vi "PH_Timing.get Timing Mode.vi"(0 "i ref in":refnum<vi>, 5 "error in":errorcluster) -> (14 "i ref out":refnum<vi>, 19 "error out":errorcluster)   [LabVIEW 2014, in "PH_Timing.lvlib"]
doc: "This VI calculates the information concerning the timing mode, writes them to own attributtes and publishes the information."
uses:
  PH_Timing.lvlib
  lib.lib/DimLVEvent/LVDimInterface/LVDimInterface.lvlib
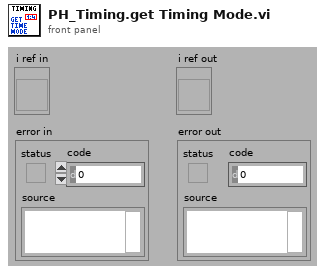
[diagram p1: front panel]
types:
  T1 = typedef "PH_Timing.lvlib/PH_Timing.i attribute.ctl" = cluster{"Sequencer":cluster{"linked?":bool, "Proc State":string, "Ref State":refnum<vi>}, "Gate Generator":cluster{"GD":cluster{"Device Status":T2, "linked?":bool}, "Settings":T3, "GUI Ref":refnum<vi>}, "Interlock Bypass":cluster{"Instancename":string, "Switch linked?":bool, "Device Status":T2, "Ref Status":refnum<vi>}, "Roughtuner":cluster{"Settings":T4, "GUI Ref":refnum<vi>, "GD":cluster{"Device Status":T2, "linked?":bool}}, "0,5Hz Gater":cluster{"Settings":T5, "GUI Ref":refnum<vi>, "GD":cluster{"Device Status":T2, "linked?":bool}}, "Slow Trigger":cluster{"Settings":T6, "GUI Ref":refnum<vi>, "Service ID Delay":i32, "Service ID Ext Trig":i32, "Wanted Settings":T6}, "Timing Mode":cluster{"Mode":T7, "GUI Ref":refnum<vi>, "Service ID T2":i32, "Service ID Mode":i32, "Wanted Mode":T7}, "ns Generator":cluster{"Settings":T8, "ns Generator Settings":refnum<vi>, "GD":cluster{"Device Status":T2, "linked?":bool}}, "Phase FEs":cluster{"Settings":T11, "GUI Ref":refnum<vi>, "Service ID Phase":i32, "Wanted Settings":T11}, "GD GUI Refs":refnum<vi>[], "Heads":T12[], "GUI Ref Delete":refnum<vi>}
  T2 = typedef "PH_StatusHandler.lvlib/PH_StatusHandler.Status.ctl" = i16
  T3 = typedef "PH_Timing.lvlib/PH_Timing.GateGen.ctl" = cluster{"Instance":string, "Channel Gate":i32, "Channel T2":i32, "Width Gate":dbl, "Width T2":dbl, "Delay Gate":dbl, "Delay T2":dbl, "Gate activ":bool, "T2 activ":bool, "System Mode":enum16{"Normal", "Single", "Burst", "Duty Cycle"}}
  T4 = typedef "PH_Timing.lvlib/PH_Timing.Roughtuner.ctl" = cluster{"Instance":string, "Phase PHELIX / UNILAC":cluster{"Channel":u16, "relative to":u16, "Delay [ms]":dbl}, "Pulse Length":cluster{"Channel":u16, "relative to":u16, "Delay [ms]":dbl}, "Trigger":cluster{"externally?":bool, "Rate [Hz]":dbl}}
  T5 = typedef "PH_Timing.lvlib/PH_Timing.0.5HzGater.ctl" = cluster{"Instance":string, "Channel ns FE Delay":i32, "Channel 0.5Hz":i32, "Width ns FE Delay":dbl, "Width 0.5Hz":dbl, "Delay ns FE Delay":dbl, "Delay 0.5Hz":dbl, "ns FE Delay active":bool, "0.5Hz activ":bool, "ns FE Delay inverted":bool, "0.5Hz inverted":bool}
  T6 = typedef "PH_Timing.lvlib/PH_Timing.Slow Trigger Settings.ctl" = cluster{"Delay":dbl, "externally triggered?":bool}
  T7 = typedef "PH_Timing.lvlib/PH_Timing.Timing Mode.ctl" = cluster{"T2":i16, "Modeselector":enum32{"10 Hz", "0.5 Hz", "Shot"}}
  T8 = typedef "PH_Timing.lvlib/PH_Timing.ns Generator.ctl" = cluster{"Instance":string, "Phase fs / ns FE":cluster{"Channel":T9, "Settings":T10}}
  T9 = typedef "Stanford Research DG645 - Driver.lvlib/Channel.ctl" = i32
  T10 = typedef "PH_SRDG645.lvlib/PH_SRDG645.Channel Settings.ctl" = cluster{"Delay [s]":dbl, "relative to":i32}
  T11 = typedef "PH_Timing.lvlib/PH_Timing.Phase FEs.ctl" = cluster{"Phase":dbl}
  T12 = typedef "PH_Timing.lvlib/PH_Timing.PU Data.ctl" = cluster{"linked?":bool, "Data":T13, "GD":cluster{"Device Status":T2, "linked?":bool}, "GUI Ref":refnum<vi>, "PU":T14}
  T13 = typedef "PH_Timing.lvlib/PH_Timing.PU Info.ctl" = cluster{"Act CH?":bool, "GD":string, "CH":i32, "Delay":dbl, "active":bool, "in Use?":bool}
  T14 = typedef "PH_PP_Common.lvlib/PH_PP_Common.PUs.ctl" = enum16{"no Info", "PA-19mm-1", "PA-19mm-2", "PA-45mm-PILC", "PA-45mm-MAIN", "MA-PU-1", "MA-PU-2", "MA-PU-3", "MA-PU-4", "MA-PU-5", "MA-PU-6", "MA-FR", "MA-PILC", "PA-45mm-DP"}
  T15 = enum16{"Normal", "Single", "Burst", "Duty Cycle"}
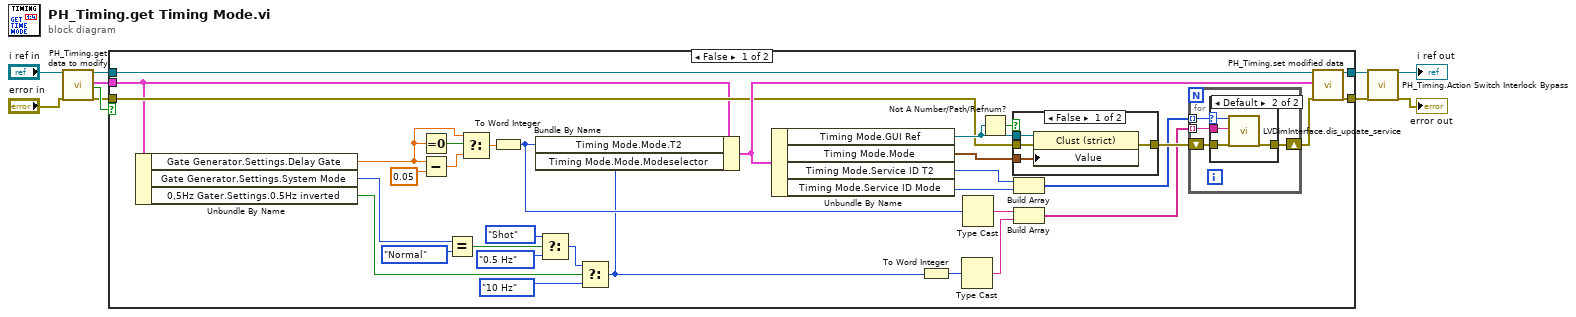
[diagram p0: block diagram]
diagram:
  n1 = call "PH_Timing.get data to modify.vi"("i ref in"="i ref in", "error in (no error)"="error in") -> ("i ref out"=w6:refnum<vi>, "i attribute"=w9:T1, "timed out"=w10:bool, "error out"=w8:errorcluster)  [unwired: 14 in]
  n2 = case shown="False" w10 {
    tunnel: w6 -> [w43 w59]
    tunnel: [w42 w59] -> w3
    tunnel: w8 -> [w35 w58]
    tunnel: [w41 w58] -> w1
    tunnel: w9 -> [w34 _]
    frame False {
      n3 = Unbundle By Name(w34) -> ("Gate Generator.Settings.Delay Gate"=w21:dbl, "Gate Generator.Settings.System Mode"=w16:T15, "0,5Hz Gater.Settings.0.5Hz inverted"=w19:bool)
      n4 = Equal To 0?(x=w21) -> (x = 0?=w25:bool)
      n5 = Subtract(x=w21, y=0.05) -> (x-y=w23:dbl)
      n6 = Equal?(x=w16, y=T15."Normal") -> (x = y?=w14:bool)
      n7 = Select(t=w21, s=w25, f=w23) -> (s? t:f=w22:dbl)
      n8 = To Word Integer(number=w22) -> (16bit integer=w20:i16)
      n9 = Select(t=enum32{"10 Hz", "0.5 Hz", "Shot"}."Shot" ("Timing Mode.Mode.Modeselector"), s=w14, f=enum32{"10 Hz", "0.5 Hz", "Shot"}."0.5 Hz" ("Timing Mode.Mode.Modeselector")) -> (s? t:f=w12:enum32{"10 Hz", "0.5 Hz", "Shot"})
      n10 = Select(t=w12, s=w19, f=enum32{"10 Hz", "0.5 Hz", "Shot"}."10 Hz" ("Timing Mode.Mode.Modeselector")) -> (s? t:f=w17:enum32{"10 Hz", "0.5 Hz", "Shot"})
      n11 = Bundle By Name(cluster=w34, "Timing Mode.Mode.T2"=w20, "Timing Mode.Mode.Modeselector"=w17) -> (w40:T1)
      n12 = Unbundle By Name(w40) -> ("Timing Mode.GUI Ref"=w38:refnum<vi>, "Timing Mode.Mode"=w37:T7, "Timing Mode.Service ID T2"=w33:i32, "Timing Mode.Service ID Mode"=w32:i32)
      n13 = To Word Integer(number=w17) -> (16bit integer=w31:i16)
      n14 = Type Cast(x=w31) -> (*(type *) &x=w29:string)  [unwired: 1 in]
      n15 = Type Cast(x=w20) -> (*(type *) &x=w30:string)  [unwired: 1 in]
      n16 = Not A Number/Path/Refnum?(number/path/refnum=w38) -> (NaN/Path/Refnum?=w39:bool)
      n17 = case shown="False" w39 {
        tunnel: [w56 w57] -> w36
        tunnel: w38 -> [w55 _]
        tunnel: w37 -> [w54 _]
        tunnel: w35 -> [w53 w57]
        frame False {
          n18 = property class="Clust (strict)"(reference=w55, error in=w53, "Value"=w54) -> (error out=w56:errorcluster)  [unwired: 1 out]
        }
        frame True {
        }
      }
      n19 = Build Array(w33, w32) -> (w26:i32[])
      n20 = Build Array(w30, w29) -> (w27:string[])
      n21 = for {
        tunnel: w26 -> [w46] mode=indexing
        tunnel: w27 -> [w44] mode=indexing
        shift-right: [w45] -> w28
        shift-left: w36 -> [w47]
        n22 = case shown="Default" w46 {
          selector: w46 -> [_ w50]
          tunnel: [w48 w51] -> w45
          tunnel: w47 -> [w48 w52]
          tunnel: w44 -> [_ w49]
          frame -1 {
          }
          frame Default {
            n23 = call "LVDimInterface.dis_update_service.vi"("my_serviceID"=w50, "data"=w49, "error in (no error)"=w52) -> ("error out"=w51:errorcluster)  [unwired: 14 in, 2 out]
          }
        }
      }
      n24 = call "PH_Timing.set modified data.vi"("i ref in"=w43, "i attribute"=w40, "error in (no error)"=w28) -> ("i ref out"=w42:refnum<vi>, "error out"=w41:errorcluster)  [unwired: 15 in]
    }
    frame True {
    }
  }
  n25 = call "PH_Timing.Action Switch Interlock Bypass.vi"("i ref in"=w3, "error in (no error)"=w1) -> ("i ref out"=→"i ref out":refnum<vi>, "error out"=→"error out":errorcluster)  [unwired: 16 in]
